vi "Nodos de control.vi"() -> ()   [LabVIEW 2020]
panel:
  in  "y":bool
  out "Fuera de rango":bool
  in  "Límite Muestreo":i32
  out "No. Muestreo":i32
  in  "Límite superior":dbl
  out "Temperatura":cluster{dbl, "Límite superior":dbl}(graph)
  out "String":string
  out "String 2":string
  in  "Numeric":dbl
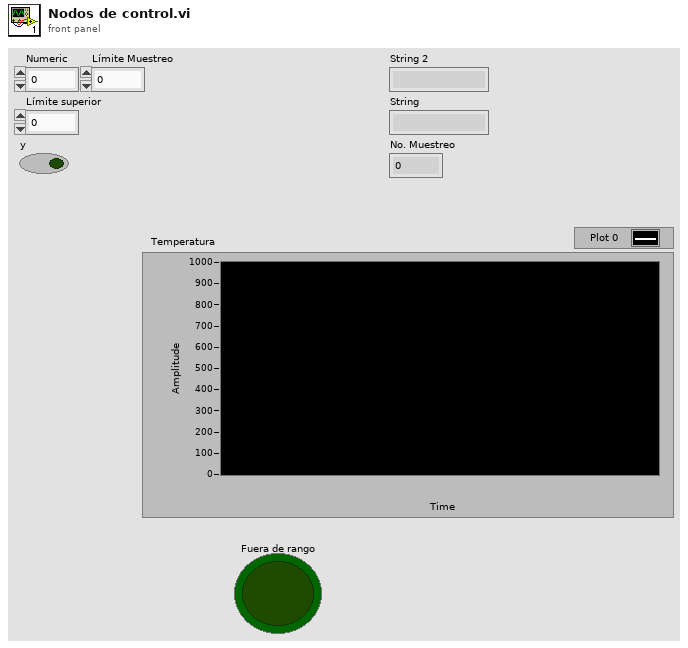
[diagram p1: front panel]
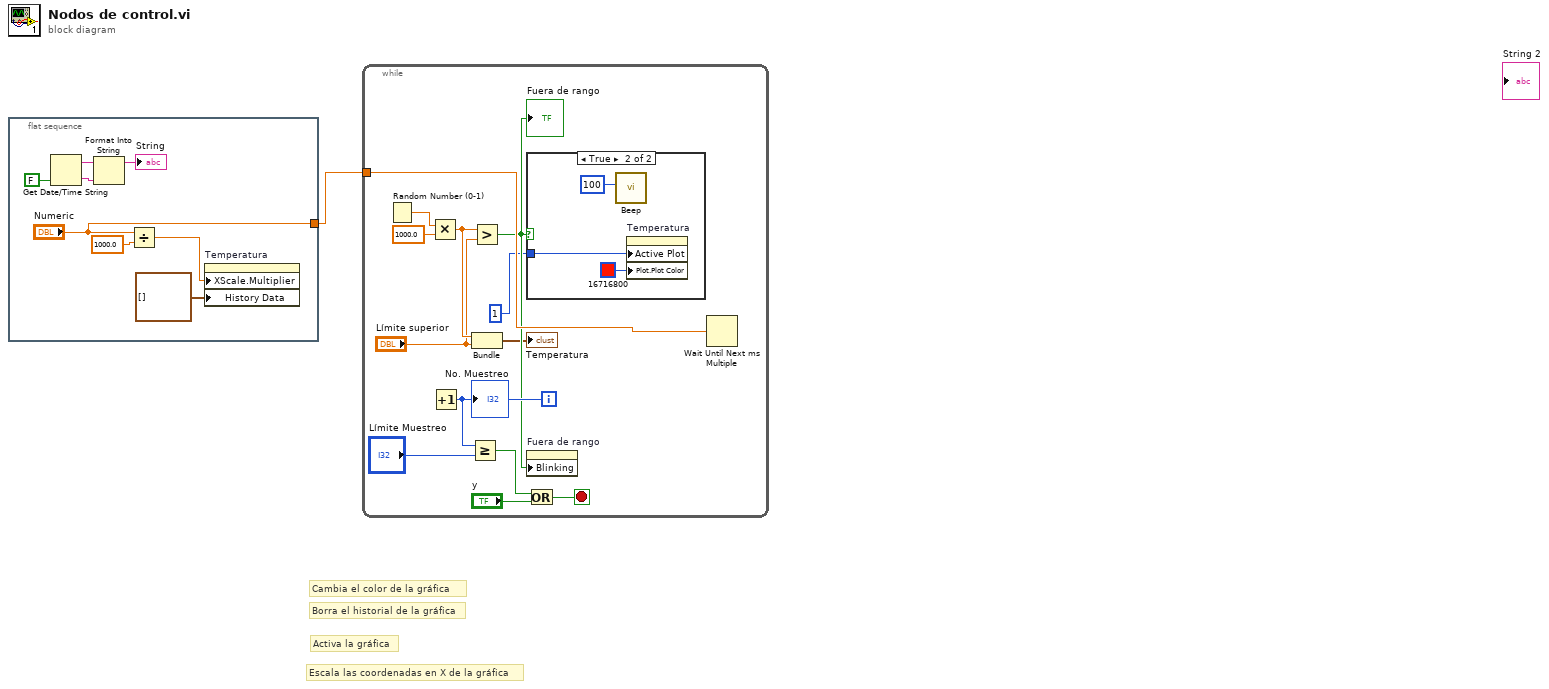
[diagram p0: block diagram]
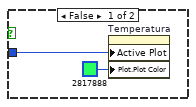
[diagram p2: hidden frame]
diagram:
  # "Escala las coordenadas en X de la gráfica"
  # "Activa la gráfica"
  # "Cambia el color de la gráfica"
  # "Borra el historial de la gráfica"
  n1 = flat-sequence {
    tunnel: ["Numeric"] -> w1
    frame #0 {
      n2 = Get Date/Time String(want seconds? (F)=FALSE) -> (date string=w7:string, time string=w6:string)  [unwired: 2 in]
      n3 = Format Into String(initial string=w7, w6) -> (resulting string=→"String":string)  [unwired: 2 in, 1 out]
      n4 = Divide(x="Numeric", y=1000.0 ("Numeric")) -> (x/y=w4:dbl)
      n5 = property on="Temperatura" class="WFChart (strict)"("XScale.Multiplier"=w4, "History Data"=cluster{dbl, "Límite superior":dbl}[] []) -> ()  [unwired: 2 in, 2 out]
    }
  }
  n6 = while {
    tunnel: w1 -> [w23]
    i -> [w16]
    stop <- w18 stop-if-true
    n7 = Random Number (0-1)() -> (number: 0 to 1=w22:dbl)
    n8 = Multiply(x=w22, y=1000.0 ("Numeric")) -> (x*y=w20:dbl)
    n9 = Increment(x=w16) -> (x+1=w15:i32)
    "No. Muestreo" <- w15
    n10 = Greater Or Equal?(x=w15, y="Límite Muestreo") -> (x >= y?=w17:bool)
    n11 = Greater?(x=w20, y="Límite superior") -> (0:w13:bool)
    "Fuera de rango" <- w13
    n12 = Bundle(w20, "Límite superior"="Límite superior") -> (→"Temperatura":cluster{dbl, "Límite superior":dbl})  [unwired: 1 in]
    n13 = case shown="True" w13 {
      tunnel: 1 -> [w25 w26]
      frame False {
        n14 = property on="Temperatura" class="WFChart (strict)"("Active Plot"=w25, "Plot.Plot Color"=u32 2817888) -> ()  [unwired: 2 in, 2 out]
      }
      frame True {
        n15 = call <vilib>:"Beep.vi"("duration (msec)"=100) -> ()  [unwired: 11 in]
        n16 = property on="Temperatura" class="WFChart (strict)"("Active Plot"=w26, "Plot.Plot Color"=u32 16716800) -> ()  [unwired: 2 in, 2 out]
      }
    }
    n17 = property on="Fuera de rango" class="Bool (strict)"("Blinking"=w13) -> ()  [unwired: 2 in, 2 out]
    n18 = Or(x=w17, y="y") -> (x .or. y?=w18:bool)
    n19 = Wait Until Next ms Multiple(millisecond multiple=w23) -> ()  [unwired: 1 out]
  }
